vi "R2_Data Collection.vi"() -> ()   [LabVIEW 2016]
uses:
  R2 Reactor Status v1.ctl
  <vilib>/Platform/TimedLoop/XDataNode/timing_clust.ctl
  <vilib>/Platform/TimedLoop/XDataNode/nitl_modes.ctl
  <vilib>/Platform/TimedLoop/XDataNode/wakeup.ctl
  R2 Pump Manual Control.ctl
  R2 DO Manual Control.ctl
  R2 pH Manual Control.ctl
  <vilib>/Platform/TimedLoop/XDataNode/XDataNode.xnode
  <vilib>/Platform/TimedLoop/XDataNode/XDNodeRunTimeDep.lvlib
  <vilib>/ptbypt/NI_PtbyPt.lvlib
  R2Variables.lvlib
panel:
  out "Numeric":i32
  out "Reactor 2 Status 2":T1
  out "N2 and Air Flow":T2(graph)
  out "pH and DO":T2(graph)
  # "Click to stop all while loops and turn off all pumps/valves."
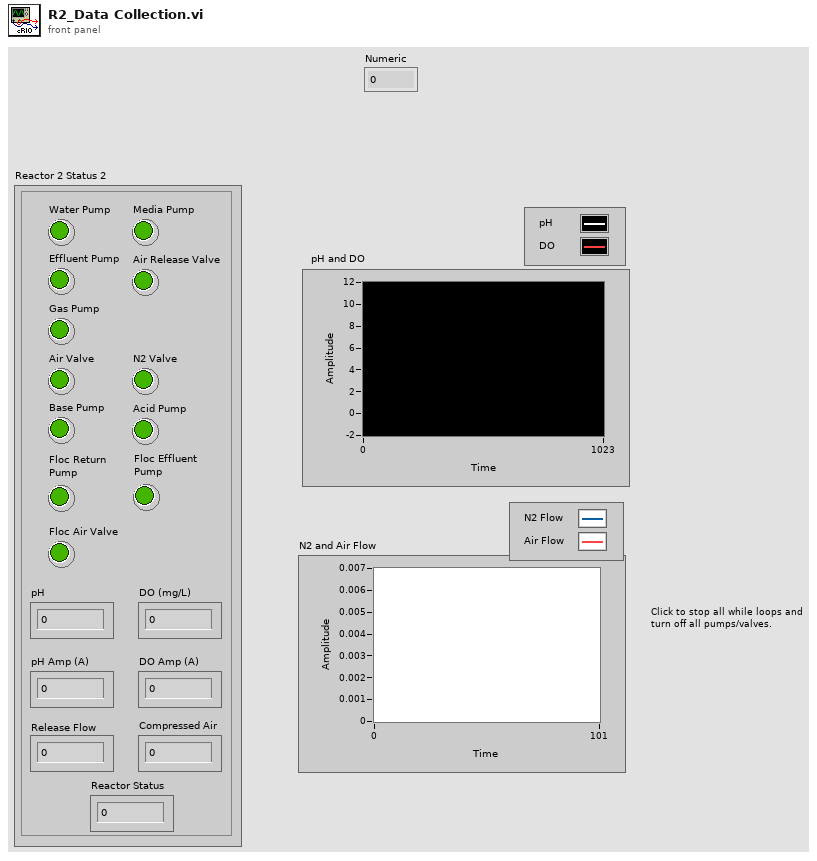
[diagram p1: front panel]
types:
  T1 = typedef "R2Variables.lvlib/R2 Reactor Status v1.ctl" = cluster{"Water Pump":bool, "Media Pump":bool, "Effluent Pump":bool, "Base Pump":bool, "Gas Pump":bool, "Acid Pump":bool, "Air Release Valve":bool, "N2 Valve":bool, "pH":dbl, "DO (mg/L)":dbl, "pH Amp (A)":dbl, "DO Amp (A)":dbl, "Release Flow":dbl, "Compressed Air":dbl, "Reactor Status":sgl, "Air Valve":bool, "Floc Return \nPump":bool, "Floc Effluent\nPump ":bool, "Floc Air Valve":bool}
  T2 = cluster{"[0]":dbl, "[1]":dbl, "[2]":dbl, "[3]":dbl, "[4]":dbl, "[5]":dbl, "[6]":dbl, "[7]":dbl, "[8]":dbl}
  T3 = typedef "R2Variables.lvlib/R2 Pump Manual Control.ctl" = cluster{"Water Pump":bool, "Effluent Pump":bool, "Media Pump":bool, "Gas Pump":bool, "Air Release Valve":bool, "Floc Effluent Pump":bool, "Floc Return Pump":bool, "Floc Air Valve":bool}
  T4 = typedef "R2Variables.lvlib/R2 DO Manual Control.ctl" = cluster{"Air Valve":bool, "N2 Valve":bool}
  T5 = typedef "R2Variables.lvlib/R2 pH Manual Control.ctl" = cluster{"Acid Pump":bool, "Base Pump":bool}
  T6 = typedef "XDNodeRunTimeDep.lvlib/timing_clust.ctl" = cluster{"Expected End [f-1]":u64, "Actual End [f-1]":u64, "Finished Late? [f-1]":bool, "Expected End [i-1]":u64, "Actual End [i-1]":u64, "Finished Late? [i-1]":bool, "Expected Start [i]":u64, "Actual Start [i]":u64, "Expected Start [f]":u64, "Actual Start [f]":u64, "Source Name":string, "Structure Name":string, "Period":i64, "Deadline":i64, "Offset":i64, "Start":i64, "Priority":i32, "Timeout":i32, "Mode":T7, "Wakeup Reason":T8, "Error":errorcluster, "Source Type":string, "Secondary Source Type":string, "Global End Time":u64, "Global Start Time":u64, "Frame Duration":u64, "Iteration Duration":u64, "Assigned CPU":i32, "I/O Scan Engine Mode":u32}
  T7 = typedef "XDNodeRunTimeDep.lvlib/nitl_modes.ctl" = enum32{"No Change", "Process missed periods, maintain original phase", "Discard missed periods, maintain original phase", "Process missed periods, ignore original phase", "Discard missed periods, ignore original phase"}
  T8 = typedef "XDNodeRunTimeDep.lvlib/wakeup.ctl" = enum32{"Normal", "Aborted", "Asynchronous wakeup", "Timing source error", "Timed loop error", "Timeout"}
  T9 = cluster{"Array of Double[0]":dbl, "Array of Double[1]":dbl, "Array of Double[2]":dbl, "Array of Double[3]":dbl, "Array of Double[4]":dbl, "Array of Double[5]":dbl, "Array of Double[6]":dbl, "Array of Double[7]":dbl, "Array of Double[8]":dbl}
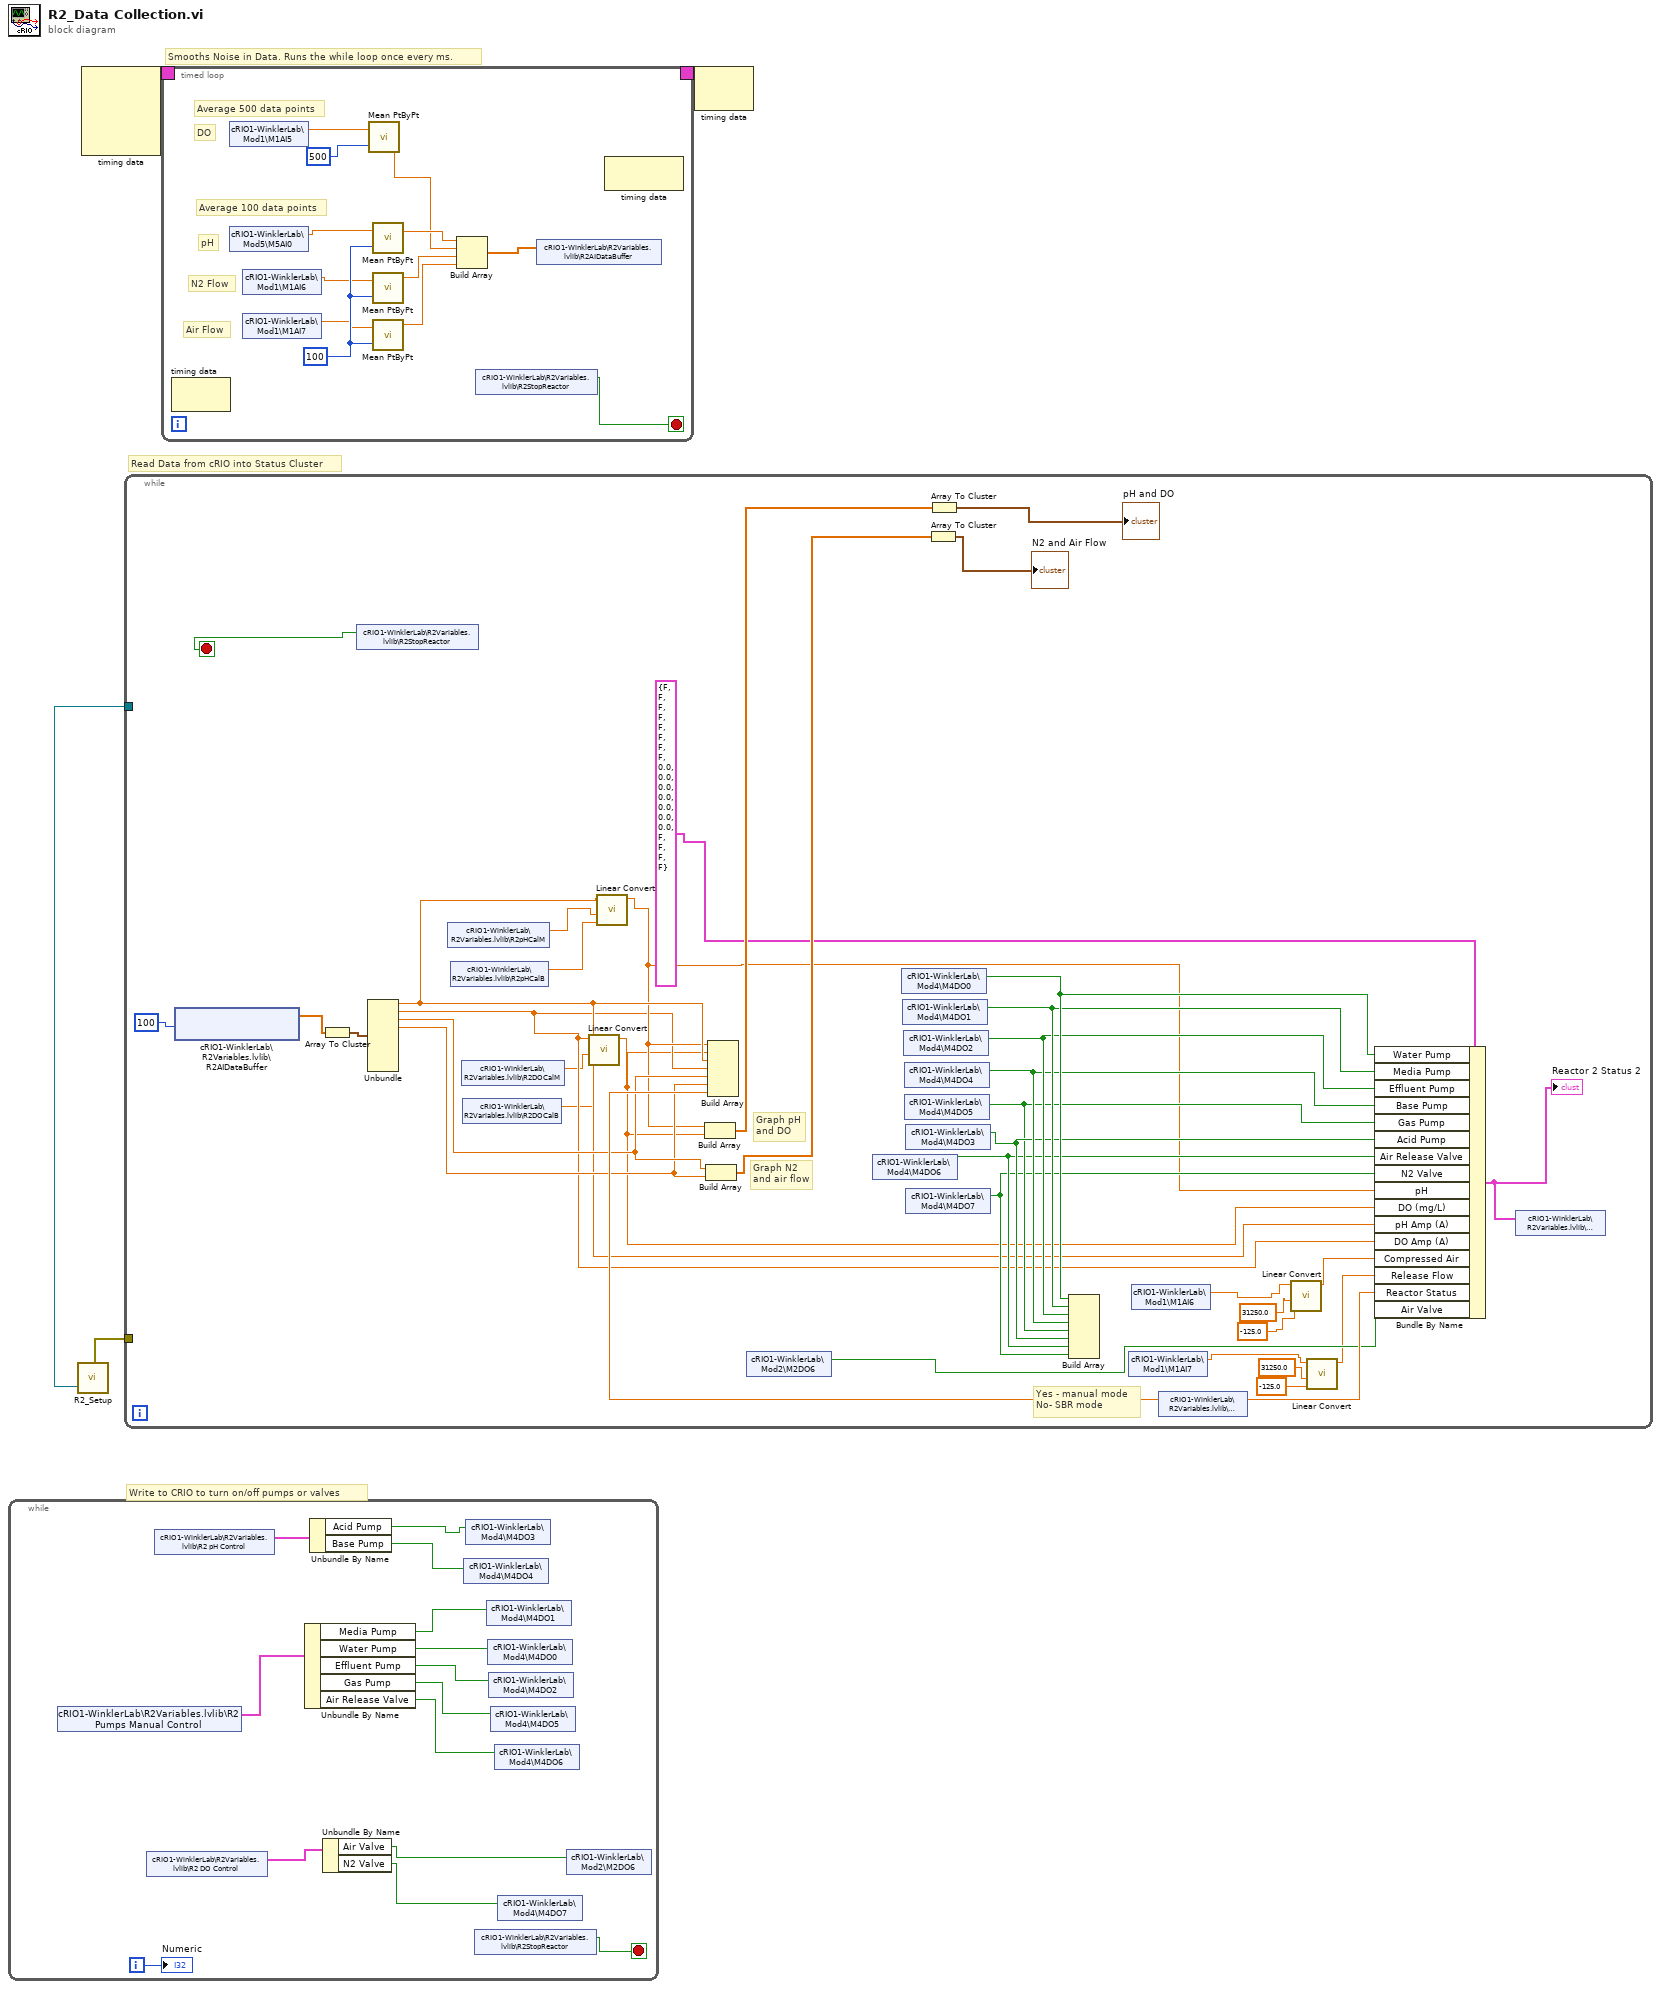
[diagram p0: block diagram]
diagram:
  # "Smooths Noise in Data. Runs the while loop once every ms."
  # "Write to CRIO to turn on/off pumps or valves"
  # "Read Data from cRIO into Status Cluster"
  n1 = while {
    i -> [w6]
    stop <- w5 stop-if-true
    n2 = shared-variable "cRIO1-WinklerLab\\R2Variables.lvlib\\R2 Pumps Manual Control"() -> (w10:T3)  [unwired: 1 in, 1 out]
    n3 = shared-variable "cRIO1-WinklerLab\\R2Variables.lvlib\\R2 DO Control"() -> (w9:T4)  [unwired: 1 in, 1 out]
    n4 = shared-variable "cRIO1-WinklerLab\\R2Variables.lvlib\\R2 pH Control"() -> (w18:T5)  [unwired: 1 in, 1 out]
    n5 = Unbundle By Name(w10) -> ("Media Pump"=w15:bool, "Water Pump"=w14:bool, "Effluent Pump"=w13:bool, "Gas Pump"=w12:bool, "Air Release Valve"=w11:bool)
    n6 = Unbundle By Name(w18) -> ("Acid Pump"=w17:bool, "Base Pump"=w16:bool)
    n7 = Unbundle By Name(w9) -> ("Air Valve"=w7:bool, "N2 Valve"=w8:bool)
    n8 = shared-variable "cRIO1-WinklerLab\\Mod4\\M4DO4"(w16) -> ()  [unwired: 1 in, 1 out]
    n9 = shared-variable "cRIO1-WinklerLab\\Mod4\\M4DO3"(w17) -> ()  [unwired: 1 in, 1 out]
    n10 = shared-variable "cRIO1-WinklerLab\\R2Variables.lvlib\\R2StopReactor"() -> (w5:bool)  [unwired: 1 in, 1 out]
    n11 = shared-variable "cRIO1-WinklerLab\\Mod4\\M4DO1"(w15) -> ()  [unwired: 1 in, 1 out]
    n12 = shared-variable "cRIO1-WinklerLab\\Mod4\\M4DO0"(w14) -> ()  [unwired: 1 in, 1 out]
    n13 = shared-variable "cRIO1-WinklerLab\\Mod4\\M4DO2"(w13) -> ()  [unwired: 1 in, 1 out]
    n14 = shared-variable "cRIO1-WinklerLab\\Mod4\\M4DO5"(w12) -> ()  [unwired: 1 in, 1 out]
    n15 = shared-variable "cRIO1-WinklerLab\\Mod4\\M4DO6"(w11) -> ()  [unwired: 1 in, 1 out]
    n16 = shared-variable "cRIO1-WinklerLab\\Mod4\\M4DO7"(w8) -> ()  [unwired: 1 in, 1 out]
    n17 = shared-variable "cRIO1-WinklerLab\\Mod2\\M2DO6"(w7) -> ()  [unwired: 1 in, 1 out]
    "Numeric" <- w6
  }
  n18 = call "R2_Setup.vi"() -> ("tdms file out"=w2:refnum<k34>, "error out"=w1:errorcluster)  [unwired: 10 in]
  n19 = node-c288() -> (w4:T6)  [unwired: 4 in]
  n20 = while {
    tunnel: w1 -> [_]
    tunnel: w2 -> [_]
    stop <- w53 stop-if-true
    # "Graph N2 and air flow"
    # "Yes - manual mode\nNo- SBR mode"
    # "Graph pH and DO"
    n21 = shared-variable "cRIO1-WinklerLab\\R2Variables.lvlib\\R2AIDataBuffer"(u32 100 ("milliseconds to wait")) -> (w42:dbl[])  [unwired: 1 in, 2 out]
    n22 = Array To Cluster(array=w42) -> (cluster=w56:T9)
    n23 = shared-variable "cRIO1-WinklerLab\\R2Variables.lvlib\\R2StopReactor"() -> (w53:bool)  [unwired: 1 in, 1 out]
    n24 = Unbundle(w56) -> ("Array of Double[0]"=w26:dbl, "Array of Double[1]"=w22:dbl, "Array of Double[2]"=w41:dbl, "Array of Double[3]"=w40:dbl)  [unwired: 5 out]
    n25 = shared-variable "cRIO1-WinklerLab\\R2Variables.lvlib\\R2pHCalM"() -> (w25:dbl)  [unwired: 1 in, 1 out]
    n26 = shared-variable "cRIO1-WinklerLab\\R2Variables.lvlib\\R2pHCalB"() -> (w24:dbl)  [unwired: 1 in, 1 out]
    n27 = shared-variable "cRIO1-WinklerLab\\R2Variables.lvlib\\R2DOCalM"() -> (w21:dbl)  [unwired: 1 in, 1 out]
    n28 = shared-variable "cRIO1-WinklerLab\\R2Variables.lvlib\\R2DOCalB"() -> (w20:dbl)  [unwired: 1 in, 1 out]
    n29 = call "Linear Convert.vi"("Intercept"=w20, "Slope"=w21, "Signal"=w22) -> ("Result"=w19:dbl)  [unwired: 8 in]
    n30 = call "Linear Convert.vi"("Intercept"=w24, "Slope"=w25, "Signal"=w26) -> ("Result"=w23:dbl)  [unwired: 8 in]
    n31 = Build Array(w23, w19) -> (w55:dbl[])
    n32 = Build Array(w41, w40) -> (w39:dbl[])
    n33 = shared-variable "cRIO1-WinklerLab\\Mod2\\M2DO6"() -> (w35:bool)  [unwired: 1 in, 1 out]
    n34 = shared-variable "cRIO1-WinklerLab\\Mod4\\M4DO6"() -> (w46:bool)  [unwired: 1 in, 1 out]
    n35 = shared-variable "cRIO1-WinklerLab\\Mod4\\M4DO0"() -> (w52:bool)  [unwired: 1 in, 1 out]
    n36 = shared-variable "cRIO1-WinklerLab\\Mod4\\M4DO1"() -> (w51:bool)  [unwired: 1 in, 1 out]
    n37 = shared-variable "cRIO1-WinklerLab\\Mod4\\M4DO2"() -> (w50:bool)  [unwired: 1 in, 1 out]
    n38 = shared-variable "cRIO1-WinklerLab\\Mod4\\M4DO4"() -> (w49:bool)  [unwired: 1 in, 1 out]
    n39 = shared-variable "cRIO1-WinklerLab\\Mod4\\M4DO5"() -> (w47:bool)  [unwired: 1 in, 1 out]
    n40 = shared-variable "cRIO1-WinklerLab\\Mod4\\M4DO3"() -> (w48:bool)  [unwired: 1 in, 1 out]
    n41 = shared-variable "cRIO1-WinklerLab\\Mod4\\M4DO7"() -> (w45:bool)  [unwired: 1 in, 1 out]
    n42 = Array To Cluster(array=w39) -> (cluster=→"N2 and Air Flow":T2)
    n43 = Array To Cluster(array=w55) -> (cluster=→"pH and DO":T2)
    n44 = Build Array(w52, w51, w50, w49, w47, w48, w46, w45) -> ()  [unwired: 1 out]
    n45 = shared-variable "cRIO1-WinklerLab\\Mod1\\M1AI7"() -> (w30:dbl)  [unwired: 1 in, 1 out]
    n46 = shared-variable "cRIO1-WinklerLab\\Mod1\\M1AI6"() -> (w34:dbl)  [unwired: 1 in, 1 out]
    n47 = shared-variable "cRIO1-WinklerLab\\R2Variables.lvlib\\R2Phase"() -> (w44:dbl)  [unwired: 1 in, 1 out]
    n48 = Build Array(w23, w19, w26, w22, w41, w40, w44) -> ()  [unwired: 1 out]
    n49 = call "Linear Convert.vi"("Intercept"=-125.0, "Slope"=31250.0, "Signal"=w34) -> ("Result"=w31:dbl)  [unwired: 8 in]
    n50 = call "Linear Convert.vi"("Intercept"=-125.0, "Slope"=31250.0, "Signal"=w30) -> ("Result"=w27:dbl)  [unwired: 8 in]
    n51 = Bundle By Name(cluster=T1 {"Water Pump"=FALSE, "Media Pump"=FALSE, "Effluent Pump"=FALSE, "Base Pump"=FALSE, "Gas Pump"=FALSE, "Acid Pump"=FALSE, "Air Release Valve"=FALSE, "N2 Valve"=FALSE, "pH"=0.0, "DO (mg/L)"=0.0, "pH Amp (A)"=0.0, "DO Amp (A)"=0.0, "Release Flow"=0.0, "Compressed Air"=0.0, "Reactor Status"=0.0, "Air Valve"=FALSE, "Floc Return \nPump"=FALSE, "Floc Effluent\nPump "=FALSE, "Floc Air Valve"=FALSE} ("Reactor 2 Status"), "Water Pump"=w52, "Media Pump"=w51, "Effluent Pump"=w50, "Base Pump"=w49, "Gas Pump"=w47, "Acid Pump"=w48, "Air Release Valve"=w46, "N2 Valve"=w45, "pH"=w23, "DO (mg/L)"=w19, "pH Amp (A)"=w26, "DO Amp (A)"=w22, "Compressed Air"=w31, "Release Flow"=w27, "Reactor Status"=w44, "Air Valve"=w35) -> (w36:T1)
    "Reactor 2 Status 2" <- w36
    n52 = shared-variable "cRIO1-WinklerLab\\R2Variables.lvlib\\R2Status"(w36) -> ()  [unwired: 1 in, 1 out]
  }
  n53 = timed-loop {
    timing: w4 -> [_]
    timing-out: [_] -> w3
    stop <- w59 stop-if-true
    w64 = 100 ("sample length")
    # "Average 100 data points"
    # "Air Flow"
    # "N2 Flow"
    # "pH"
    # "DO"
    # "Average 500 data points"
    n54 = node-c288() -> ()  [unwired: 1 in, 1 out]
    n55 = shared-variable "cRIO1-WinklerLab\\Mod1\\M1AI5"() -> (w62:dbl)  [unwired: 1 in, 1 out]
    n56 = shared-variable "cRIO1-WinklerLab\\Mod5\\M5AI0"() -> (w57:dbl)  [unwired: 1 in, 1 out]
    n57 = shared-variable "cRIO1-WinklerLab\\Mod1\\M1AI6"() -> (w61:dbl)  [unwired: 1 in, 1 out]
    n58 = shared-variable "cRIO1-WinklerLab\\Mod1\\M1AI7"() -> (w60:dbl)  [unwired: 1 in, 1 out]
    n59 = call <vilib>:"Mean PtByPt.vi"("x"=w62, "sample length"=500) -> ("mean"=w67:dbl)  [unwired: 2 in, 1 out]
    n60 = call <vilib>:"Mean PtByPt.vi"("x"=w57, "sample length"=w64) -> ("mean"=w68:dbl)  [unwired: 2 in, 1 out]
    n61 = call <vilib>:"Mean PtByPt.vi"("x"=w61, "sample length"=w64) -> ("mean"=w66:dbl)  [unwired: 2 in, 1 out]
    n62 = call <vilib>:"Mean PtByPt.vi"("x"=w60, "sample length"=w64) -> ("mean"=w65:dbl)  [unwired: 2 in, 1 out]
    n63 = Build Array(w68, w67, w66, w65) -> (w58:dbl[])
    n64 = shared-variable "cRIO1-WinklerLab\\R2Variables.lvlib\\R2StopReactor"() -> (w59:bool)  [unwired: 1 in, 1 out]
    n65 = shared-variable "cRIO1-WinklerLab\\R2Variables.lvlib\\R2AIDataBuffer"(w58) -> ()  [unwired: 1 in, 1 out]
    n66 = node-c288() -> ()  [unwired: 1 in, 1 out]
  }
  n67 = node-c288(w3) -> ()  [unwired: 1 out]
